vi "Global_Joystick Write_Data.vi"() -> ()   [LabVIEW 2016, in "Controller.lvlib"]
uses:
  Controller.lvlib
panel:
  out "Joystick_SEN_POVs":i16[](array[numeric])
  out "Joystick_SEN_Buttons":bool[](array[boolean])
  out "Joystick_SEN_Axes":dbl[](array[numeric])
  # "The Names of the Data items in the Global Variable MUST describe who the Single Writer is\nNaming Convention of all Data Items is:   Lib Name_Loop Name (SM or SEN or ACT)_Data Name\nExample   Drive_ACT_X axis;  GameController_SEN_JoystickLeft;  Hopper_SM_AgitatorSpeed"
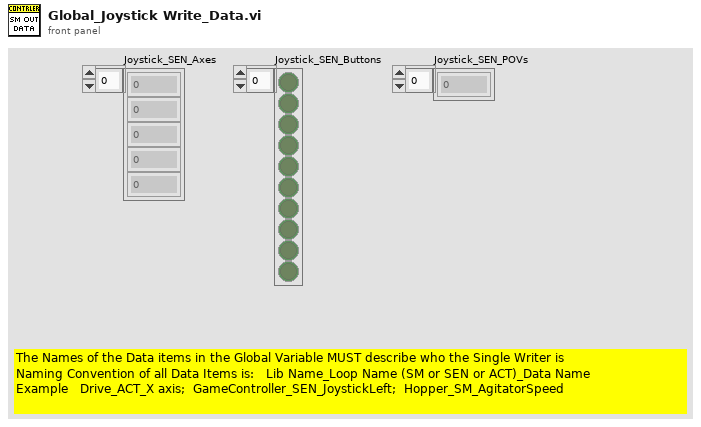
[diagram p1: front panel]
diagram:
